vi "Read (Multiple Points).vi"(0 "VISA resource name":refnum<visa-resource-name>, 5 "Timeout (10000 ms)":u32=10000, 11 "error in":errorcluster) -> (3 "Go":bool, 4 "VISA resource name out":refnum<visa-resource-name>, 6 "Measurements":dbl[](array[numeric]), 10 "Questionable Data":bool, 13 "High":bool, 14 "Low":bool, 15 "error out":errorcluster)   [LabVIEW 2017, in "ADCMT 6240.lvlib"]
doc: "Reads and returns multiple measurements from the instrument. \nUse this VI when you want to take multiple measurements using an auto trigger. \nUse the low level VIs for other triggering options."
uses:
  ADCMT 6240.lvlib
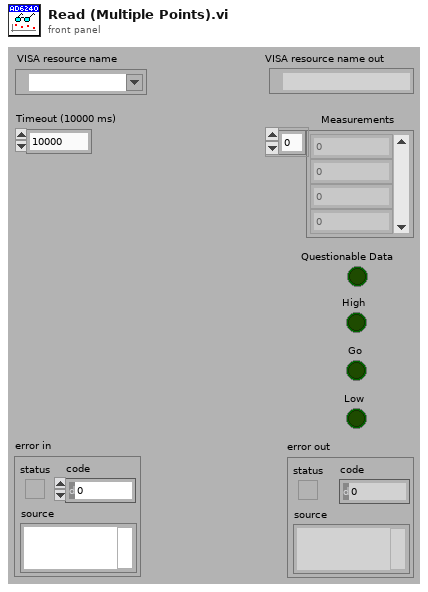
[diagram p1: front panel]
types:
  T1 = typedef "ADCMT 6240.lvlib/Extended User Data.ctl" = cluster{"Trigger Mode":u16, "Output Mode":u16, "Sample Count":i32, "Model":u16}
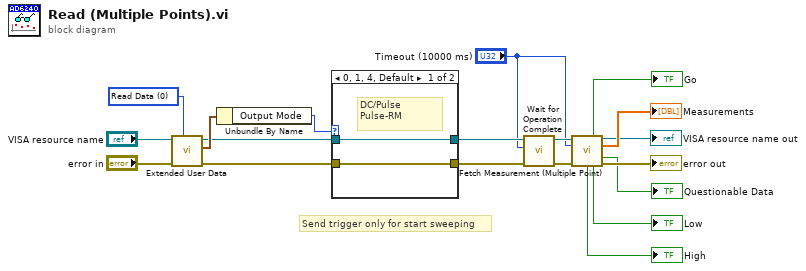
[diagram p0: block diagram]
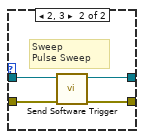
[diagram p2: hidden frame]
diagram:
  w10 = u16 0 items=["Read Data", "Write Data", "Dispose of Data"] ("Action")
  # "Send trigger only for start sweeping"
  n1 = call "Extended User Data.vi"("Action"=w10, "Error In (no error)"="error in", "VISA resource name in"="VISA resource name") -> ("Error Out"=w5:errorcluster, "User Data Out"=w11:T1, "VISA resource name out"=w6:refnum<visa-resource-name>)  [unwired: 6 in]
  n2 = Unbundle By Name(w11) -> ("Output Mode"=w9:u16)
  n3 = case shown="0, 1, 4, Default" w9 {
    tunnel: [w20 w25] -> w18
    tunnel: [w21 w24] -> w17
    tunnel: w6 -> [w21 w23]
    tunnel: w5 -> [w20 w22]
    frame 0, 1, 4, Default {
      # "DC/Pulse\nPulse-RM"
    }
    frame 2, 3 {
      # "Sweep\nPulse Sweep"
      n4 = call "Send Software Trigger.vi"("error in (no error)"=w22, "VISA resource name"=w23) -> ("error out"=w25:errorcluster, "VISA resource name out"=w24:refnum<visa-resource-name>)  [unwired: 8 in]
    }
  }
  n5 = call "Wait for Operation Complete.vi"("error in (no error)"=w18, "Timeout (10000 ms)"="Timeout (10000 ms)", "VISA resource name"=w17) -> ("error out"=w15:errorcluster, "VISA resource name out"=w16:refnum<visa-resource-name>)  [unwired: 7 in]
  n6 = call "Fetch Measurement (Multiple Point).vi"("VISA resource name"=w16, "Timeout (10000 ms)"="Timeout (10000 ms)", "error in (no error)"=w15) -> ("Go"=→"Go":bool, "VISA resource name out"=→"VISA resource name out":refnum<visa-resource-name>, "Measurements"=→"Measurements":dbl[], "Questionable Data"=→"Questionable Data":bool, "High"=→"High":bool, "Low"=→"Low":bool, "error out"=→"error out":errorcluster)  [unwired: 6 in]
